vi "QDMH Main.vi"(8 "error in (no error)":errorcluster, 10 "Queue Name":string) -> (0 "error out":errorcluster)   [LabVIEW 2011]
doc: "This is a basic Queue Driven Message Handler VI. Most advanced LabVIEW programmers who code extensively in LabVIEW utilitze some variation of this VI. This is a starting point. Some key features need to be added. In particular a robust error handling routine should be added.\n\nAAL 9/09"
uses:
  Shared/QDMH Poly VIs/QDMH POLY Enqueue String.vi
panel:
  in  "New button 2":bool
  in  "New button 1":bool
  in  "Launch Dynamic":bool
  out "Message Display":string
  in  "Cancel":bool
  in  "OK":bool
  # "Note:  You must first save the VI and the VI Cluster\nin the same directory as QDMH Main.vit in order for \nthe Launch Dynamic to work."
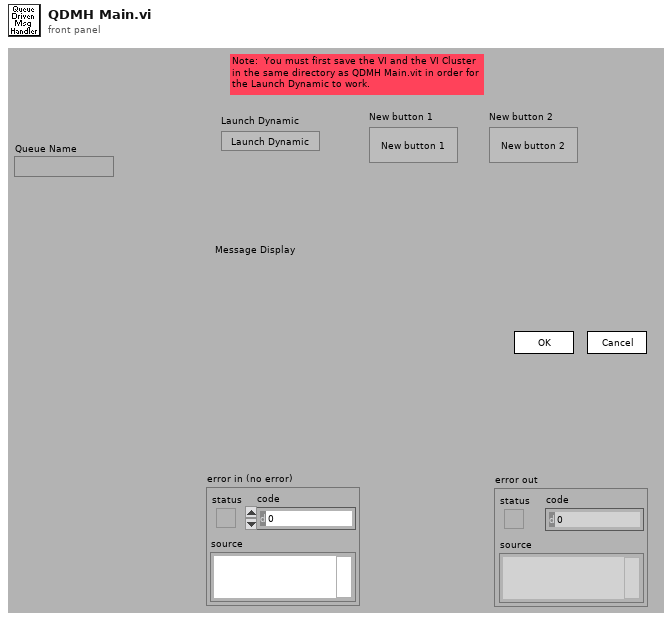
[diagram p1: front panel]
types:
  T1 = cluster{"Operator Name":string, "Current VI's Path":path, "Current VI's  Directory":path, "Queue Names":string[], "# VIs Launched":i32}
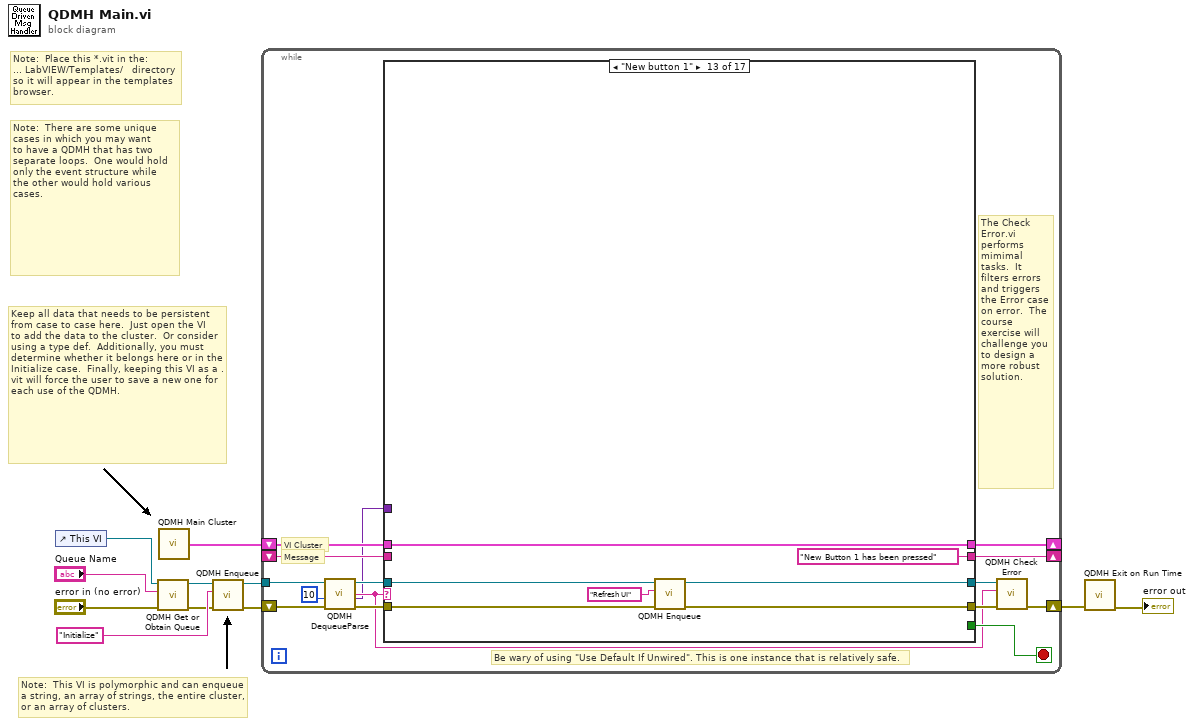
[diagram p0: block diagram]
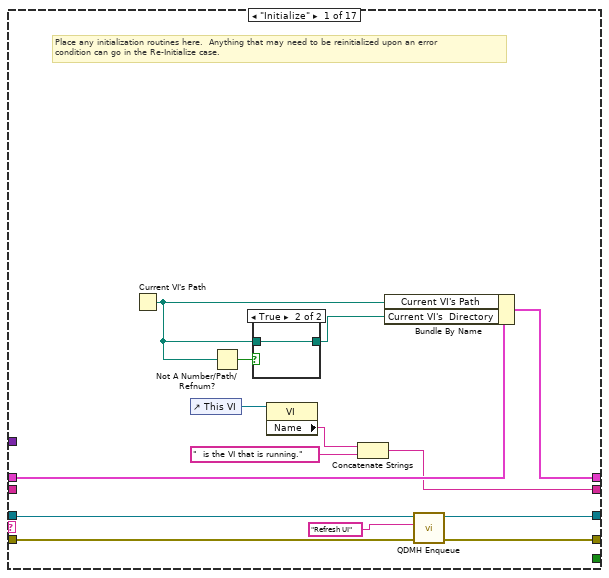
[diagram p2: hidden frame]
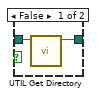
[diagram p3: hidden frame]
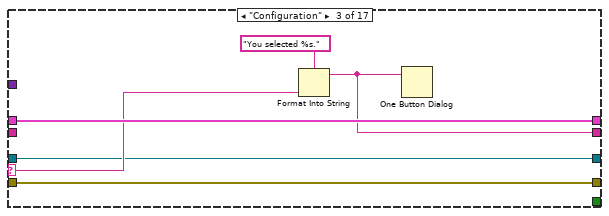
[diagram p5: hidden frame]
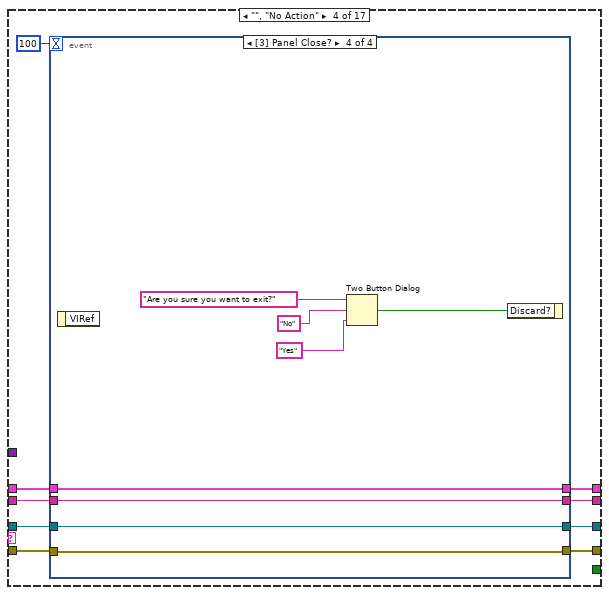
[diagram p6: hidden frame]
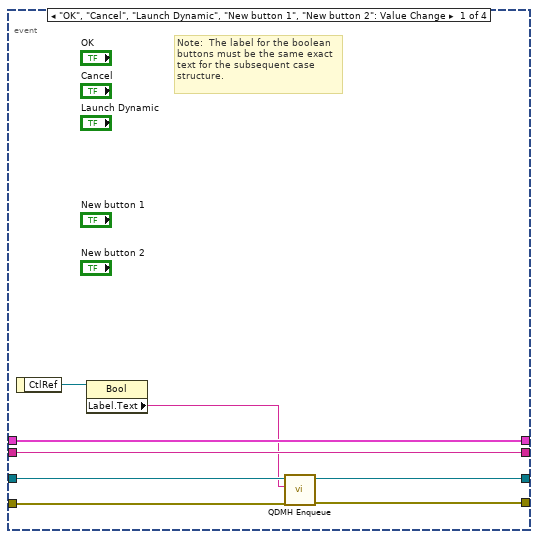
[diagram p7: hidden frame]
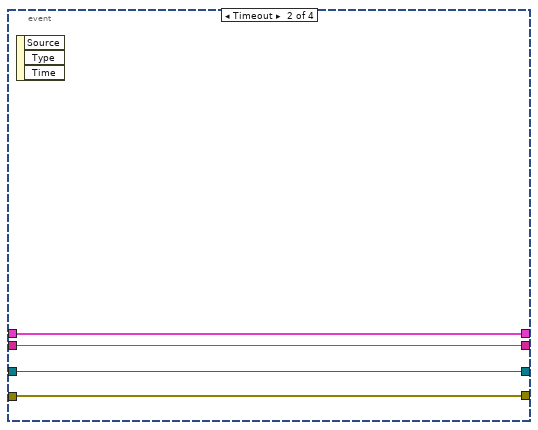
[diagram p8: hidden frame]
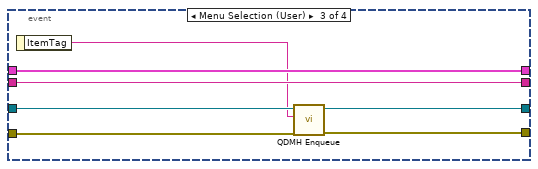
[diagram p9: hidden frame]
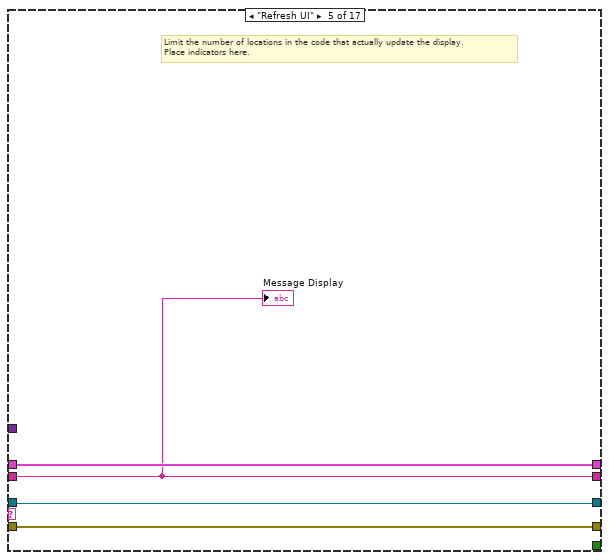
[diagram p10: hidden frame]
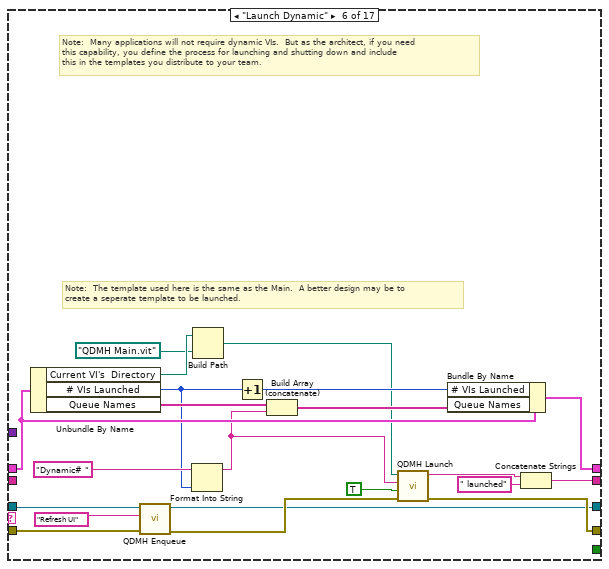
[diagram p11: hidden frame]
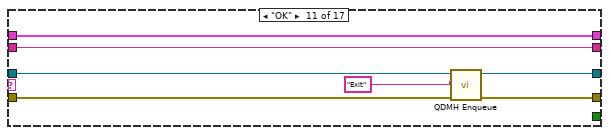
[diagram p16: hidden frame]
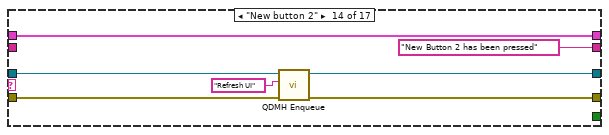
[diagram p18: hidden frame]
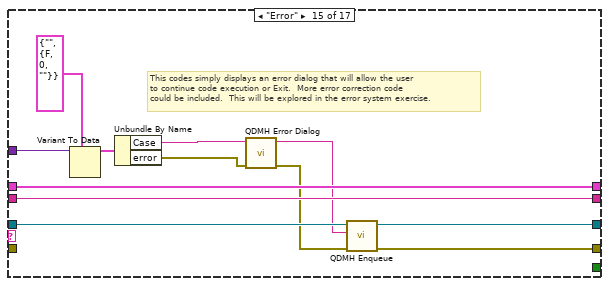
[diagram p19: hidden frame]
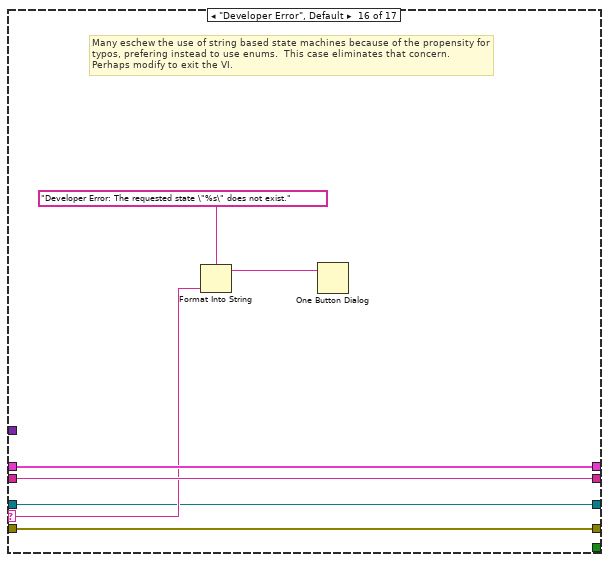
[diagram p20: hidden frame]
diagram:
  # "Note:  There are some unique\ncases in which you may want\nto have a QDMH that has two\nseparate loops.  One would hold\nonly the event structure while\nthe other would hold various \ncases."
  # "Note:  Place this *.vit in the:\n... LabVIEW/Templates/   directory\nso it will appear in the templates\nbrowser."
  # "Note:  This VI is polymorphic and can enqueue\na string, an array of strings, the entire cluster,\nor an array of clusters."
  # "Keep all data that needs to be persistent\nfrom case to case here.  Just open the VI\nto add the data to the cluster.  Or consider \nusing a type def.  Additionally, you must determine whether it belongs here or in the Initialize case.  Finally, keeping this VI as a .vit will force the user to save a new one for each use of the QDMH."
  n1 = control-ref of="This VI"() -> (w3:refnum<vi>)
  n2 = call "QDMH Get or Obtain Queue.vi"("error in (no error)"="error in (no error)", "Queue Name"="Queue Name", "VI Refnum"=w3) -> ("error out"=w6:errorcluster, "queue out"=w7:refnum<queue>)  [unwired: 7 out]
  n3 = call "QDMH Main Cluster.vi"() -> ("Cluster"=w11:T1)
  n4 = call-poly "QDMH Enqueue.vi"("error in (no error)"=w6, "State"="Initialize" ("element"), "queue"=w7) -> ("error out"=w4:errorcluster, "queue out"=w5:refnum<queue>)  [unwired: 7 out]
  n5 = while {
    tunnel: w5 -> [w21]
    shift-left: w11 -> [w22]
    shift-right: [w23] -> _
    shift-left: _ -> [w24]
    shift-right: [w25] -> _
    shift-right: [w15] -> w2
    shift-left: w4 -> [w17]
    stop <- w26 stop-if-true
    # "Be wary of using \"Use Default If Unwired\". This is one instance that is relatively safe."
    # "VI Cluster"
    # "Message"
    # "The Check Error.vi performs mimimal tasks.  It filters errors and triggers the Error case on error.  The course exercise will challenge you to design a more robust solution."
    n6 = call "QDMH DequeueParse.vi"("error in (no error)"=w17, "Timeout"=10 ("ms timeout (-1)"), "queue"=w21) -> ("error out"=w18:errorcluster, "Variant Data"=w12:variant, "State"=w13:string, "queue out"=w19:refnum<queue>)  [unwired: 5 out]
    n7 = case shown="\"New button 1\"" w13 {
      selector: w13 -> [_ _ w50 _ _ _ _ _ _ _ _ _ _ _ _ w171 _]
      tunnel: w19 -> [w36 w44 w49 w62 w91 w110 w115 w119 w123 w127 w137 w139 w146 w152 w165 w168 w181]
      tunnel: [_ _ _ _ _ _ _ _ _ _ _ _ _ _ _ _ TRUE] -> w26
      tunnel: [w34 w47 w51 w55 w92 w111 w118 w122 w126 w130 w136 w141 "New Button 1 has been pressed" "New Button 2 has been pressed" w167 w174 w183] -> w25
      tunnel: w24 -> [_ w47 _ w56 w92 _ w118 w122 w126 w130 w136 w141 _ _ w167 w174 w183]
      tunnel: [w39 w46 w53 w57 w93 w107 w117 w121 w125 w129 w135 w140 w148 w155 w166 w173 w178] -> w23
      tunnel: w22 -> [w40 w46 w53 w58 w93 w108 w117 w121 w125 w129 w135 w140 w148 w155 w166 w173 w178]
      tunnel: w18 -> [w38 w45 w48 w61 w90 w101 w116 w120 w124 w128 w134 w138 w144 w150 _ w170 w180]
      tunnel: [w37 w45 w48 w60 w90 w100 w116 w120 w124 w128 w133 w138 w143 w149 w164 w170 w175] -> w16
      tunnel: [w29 w44 w49 w54 w91 w97 w115 w119 w123 w127 w131 w139 w145 w151 w163 w168 refnum<queue> refnum ("queue out")] -> w14
      tunnel: w12 -> [_ _ _ _ _ _ _ _ _ _ _ _ _ _ w161 _ _]
      frame "Initialize" {
        # "Place any initialization routines here.  Anything that may need to be reinitialized upon an error\ncondition can go in the Re-Initialize case."
        n8 = Current VI's Path() -> (path=w27:path)
        n9 = control-ref of="This VI"() -> (w33:refnum<vi>)
        n10 = Not A Number/Path/Refnum?(number/path/refnum=w27) -> (NaN/Path/Refnum?=w28:bool)
        n11 = case shown="True" w28 {
          tunnel: w27 -> [w42 w43]
          tunnel: [w41 w43] -> w31
          frame False {
            n12 = call "UTIL Get Directory.vi"("Path In"=w42) -> ("Directory Out"=w41:path)  [unwired: 1 in, 9 out]
          }
          frame True {
          }
        }
        n13 = property class="VI"(reference=w33) -> ("Name"=w32:string)  [unwired: 1 in, 2 out]
        n14 = Concatenate Strings(w32, "  is the VI that is running." ("string")) -> (w34:string)
        n15 = Bundle By Name(cluster=w40, "Current VI's Path"=w27, "Current VI's  Directory"=w31) -> (w39:T1)
        n16 = call-poly "QDMH Enqueue.vi"("error in (no error)"=w38, "State"="Refresh UI" ("New State"), "queue"=w36) -> ("error out"=w37:errorcluster, "queue out"=w29:refnum<queue>)  [unwired: 7 out]
      }
      frame "Re-Initialize" {
        # "This case includes initialization functionality that may need to run again during the course of the VI"
      }
      frame "Configuration" {
        n17 = Format Into String(format string="You selected %s." ("Format String"), w50) -> (resulting string=w51:string)  [unwired: 2 in, 1 out]
        n18 = One Button Dialog(message=w51) -> ()  [unwired: 2 out]
      }
      frame "", "No Action" {
        n19 = event shown="[3] Panel Close?" {
          selector: _ -> [_ _ _ _]
          dyn-events: _ -> [_ _ _ _]
          timeout: 100 -> [_ _ _ _]
          tunnel: w62 -> [w69 w71 w81 w83]
          tunnel: [w68 w74 w79 w82] -> w60
          tunnel: w61 -> [w67 w74 w80 w82]
          tunnel: w58 -> [w66 w73 w78 w89]
          tunnel: [w66 w73 w78 w89] -> w57
          tunnel: w56 -> [w65 w72 w77 w88]
          tunnel: [w65 w72 w77 w88] -> w55
          tunnel: [w63 w71 w75 w83] -> w54
          event "OK", "Cancel", "Launch Dynamic", "New button 1", "New button 2": Value Change {
            # "Note:  The label for the boolean buttons must be the same exact text for the subsequent case structure."
            n20 = event-data() -> ("CtlRef"=w70:refnum<vi>)  [unwired: 1 out]
            n21 = property class="Bool"(reference=w70) -> ("Label.Text"=w64:string)  [unwired: 1 in, 2 out]
            n22 = call-poly "QDMH Enqueue.vi"("error in (no error)"=w67, "State"=w64, "queue"=w69) -> ("error out"=w68:errorcluster, "queue out"=w63:refnum<queue>)  [unwired: 7 out]
          }
          event Timeout {
            n23 = event-data() -> ()  [unwired: 4 out]
          }
          event Menu Selection (User) {
            n24 = event-data() -> ("ItemTag"=w76:string)  [unwired: 1 out]
            n25 = call-poly "QDMH Enqueue.vi"("error in (no error)"=w80, "State"=w76, "queue"=w81) -> ("error out"=w79:errorcluster, "queue out"=w75:refnum<queue>)  [unwired: 7 out]
          }
          event Panel Close? {
            n26 = event-data() -> ()  [unwired: 2 out]
            n27 = Two Button Dialog(message="Are you sure you want to exit?", 1:"Yes" ("F button name (\"Cancel\")"), 2:"No" ("T button name (\"OK\")")) -> (T button?=w84:bool)
            n28 = event-data("Discard?"=w84) -> ()  [unwired: 1 in, 1 out]
          }
        }
      }
      frame "Refresh UI" {
        # "Limit the number of locations in the code that actually update the display.\nPlace indicators here."
        "Message Display" <- w92
      }
      frame "Launch Dynamic" {
        # "Note:  The template used here is the same as the Main.  A better design may be to\ncreate a seperate template to be launched."
        # "Note:  Many applications will not require dynamic VIs.  But as the architect, if you need\nthis capability, you define the process for launching and shutting down and include\nthis in the templates you distribute to your team."
        n29 = Unbundle By Name(w108) -> ("Current VI's  Directory"=w96:path, "# VIs Launched"=w104:i32, "Queue Names"=w106:string[])
        n30 = call-poly "QDMH Enqueue.vi"("error in (no error)"=w101, "State"="Refresh UI" ("New State"), "queue"=w110) -> ("error out"=w99:errorcluster, "queue out"=w97:refnum<queue>)  [unwired: 7 out]
        n31 = Format Into String(initial string="Dynamic# ", w104) -> (resulting string=w102:string)  [unwired: 2 in, 1 out]
        n32 = Build Path(base path=w96, name or relative path=path "QDMH Main.vit" ("vi path")) -> (appended path=w94:path)
        n33 = Increment(x=w104) -> (x+1=w103:i32)
        n34 = Build Array (concatenate)(w106, w102) -> (w105:string[])
        n35 = call "QDMH Launch.vi"("error in (no error)"=w99, "Front Panel Window (Open)"=TRUE ("Front Panel Window:Open"), "Queue Name"=w102, "VI Path"=w94) -> ("error out"=w100:errorcluster, "Launched VI Name"=w113:string)  [unwired: 6 out]
        n36 = Bundle By Name(cluster=w108, "# VIs Launched"=w103, "Queue Names"=w105) -> (w107:T1)
        n37 = Concatenate Strings(w113, " launched" ("string")) -> (w111:string)
      }
      frame "Shutdown Dynamic" {
      }
      frame "Send Message to Dynamic" {
      }
      frame "Receive Message From Dynamic" {
      }
      frame "<duplicate me for new states >" {
        # "Duplicate this state for any additional states that you add."
      }
      frame "OK" {
        n38 = call-poly "QDMH Enqueue.vi"("error in (no error)"=w134, "State"="Exit" ("New State"), "queue"=w137) -> ("error out"=w133:errorcluster, "queue out"=w131:refnum<queue>)  [unwired: 7 out]
      }
      frame "Cancel" {
      }
      frame "New button 1" {
        n39 = call-poly "QDMH Enqueue.vi"("error in (no error)"=w144, "State"="Refresh UI" ("New State"), "queue"=w146) -> ("error out"=w143:errorcluster, "queue out"=w145:refnum<queue>)  [unwired: 7 out]
      }
      frame "New button 2" {
        n40 = call-poly "QDMH Enqueue.vi"("error in (no error)"=w150, "State"="Refresh UI" ("New State"), "queue"=w152) -> ("error out"=w149:errorcluster, "queue out"=w151:refnum<queue>)  [unwired: 7 out]
      }
      frame "Error" {
        # "This codes simply displays an error dialog that will allow the user\nto continue code execution or Exit.  More error correction code\ncould be included.  This will be explored in the error system exercise."
        n41 = Variant To Data(type=cluster{"Case":string, "error":errorcluster} {"Case"="", "error"={"status"=FALSE, "code"=0, "source"=""}} ("QDSM Element"), Variant=w161) -> (data=w160:cluster{"Case":string, "error":errorcluster})  [unwired: 1 in, 1 out]
        n42 = Unbundle By Name(w160) -> ("Case"=w159:string, "error"=w158:errorcluster)
        n43 = call "QDMH Error Dialog.vi"("error"=w158, "Case Error Occured"=w159) -> ("error out (no error)"=w156:errorcluster, "Case to Execute"=w157:string)  [unwired: 8 out]
        n44 = call-poly "QDMH Enqueue.vi"("error in (no error)"=w156, "State"=w157, "queue"=w165) -> ("error out"=w164:errorcluster, "queue out"=w163:refnum<queue>)  [unwired: 7 out]
      }
      frame "Developer Error", Default {
        # "Many eschew the use of string based state machines because of the propensity for\ntypos, prefering instead to use enums.  This case eliminates that concern.\nPerhaps modify to exit the VI."
        n45 = Format Into String(format string="Developer Error: The requested state \"%s\" does not exist." ("message"), w171) -> (resulting string=w169:string)  [unwired: 2 in, 1 out]
        n46 = One Button Dialog(message=w169) -> ()  [unwired: 2 out]
      }
      frame "Exit" {
        # "Note:  The release queue function has the force destroy option set to true."
        # "Place any critical clean up routines here."
        n47 = Unbundle By Name(w178) -> ("Queue Names"=w176:string[])
        n48 = Release Queue(queue=w181, force destroy? (F)=TRUE, error in (no error)=w180) -> (error out=w175:errorcluster)  [unwired: 2 out]
        n49 = for {
          tunnel: w176 -> [w188] mode=indexing
          n50 = Obtain Queue(name (unnamed)=w188, element data type=cluster{"State":string, "Variant Data":variant} {"State"="", "Variant Data"=variant} ("QDSM Element")) -> (queue out=w187:refnum<queue>)  [unwired: 3 in, 2 out]
          n51 = call-poly "QDMH Enqueue.vi"("State"="Exit" ("element"), "queue"=w187) -> ()  [unwired: 1 in, 9 out]
        }
        n52 = local write "Message Display"("") -> ()
      }
    }
    n53 = call "QDMH Check Error.vi"("error in (no error)"=w16, "Case"=w13, "queue"=w14) -> ("error out"=w15:errorcluster)  [unwired: 1 in, 7 out]
  }
  n54 = call "QDMH Exit on Run Time.vi"("error in (no error)"=w2) -> ("error out"=→"error out":errorcluster)  [unwired: 10 in]
